vi "Configure Frequency Sweep at Constant Amplitude.vi"(0 "template configuration":refnum<class "SV Signal.lvclass">, 1 "amplitude":dbl=1.0, 5 "frequency range [Hz]":cluster{"start":dbl, "stop":dbl}={"start"=10.0, "stop"=10000.0} {"stop" format="%.2f"; "start" format="%.2f"}, 7 "number of steps":i32=100 min=1, 9 "profile":enum16{"Linear", "Logarithmic"}(ring)=enum."Logarithmic", 11 "error in (no error)":errorcluster) -> (4 "signal configuration":refnum<class "SV Discrete Sweep.lvclass">, 15 "error out":errorcluster)   [LabVIEW 2017, in "SV Discrete Sweep.lvclass"]
doc: "Configures a user-defined test signal. Wire the outputs to SV Signal (waveform) VI to generate the test signal, or wire to SV Signal Property Node to configure additional parameters before wiring to the SV Signal (waveform) VI."
uses:
  <vilib>/addons/_NISVFA/_Generation/Signal Generation/SV Discrete Sweep/SV Discrete Sweep.lvclass
  C:/Program Files (x86)/National Instruments/LabVIEW 2017/vi.lib/addons/_NISVFA/_Generation/Signal Generation/SV Signal/SV Signal.lvclass
  C:/Program Files (x86)/National Instruments/LabVIEW 2017/vi.lib/addons/_NISVFA/_Generation/Signal Generation/SV Function/SV Function.lvclass
  <vilib>/addons/_NISVFA/_Generation/Signal Generation/SV Signal/SV Signal.lvclass
  <vilib>/addons/_NISVFA/_Generation/Signal Generation/SV Signal/sv_System Timing Model.ctl
  <vilib>/addons/_NISVFA/_Generation/Signal Generation/SV Discrete Sweep/SV Discrete Sweep.lvclass/SV Discrete Sweep.ctl
  <vilib>/addons/_NISVFA/_Generation/Signal Generation/SV Signal/Write System Timing Model.vi
  <vilib>/addons/_NISVFA/_Generation/Signal Generation/SV Function/Write Measurement Cycles.vi
  <vilib>/addons/_NISVFA/_Generation/Signal Generation/SV Signal/Write Sample Rate.vi
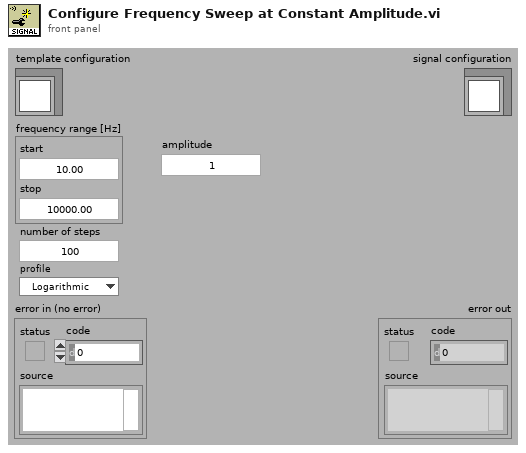
[diagram p1: front panel]
types:
  T1 = cluster{"start frequency":dbl, "stop frequency":dbl, "number of steps":i32}
  T2 = typedef "SV Signal.lvclass/sv_System Timing Model.ctl" = i64
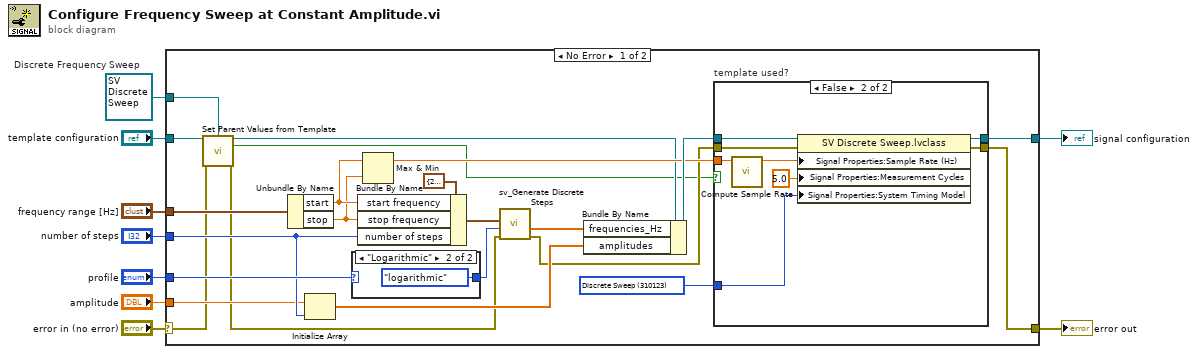
[diagram p0: block diagram]
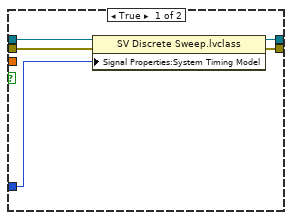
[diagram p2: hidden frame]
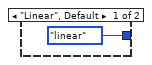
[diagram p3: hidden frame]
diagram:
  w7 = refnum<class "SV Discrete Sweep.lvclass"> refnum  # Discrete Frequency Sweep
  n1 = case shown="No Error" "error in (no error)" {
    selector: "error in (no error)" -> [w12 w48]
    tunnel: [w19 w48] -> w8
    tunnel: [w24 w49] -> w6
    tunnel: w7 -> [w14 w49]
    tunnel: "frequency range [Hz]" -> [w32 _]
    tunnel: "number of steps" -> [w27 _]
    tunnel: "profile" -> [w29 _]
    tunnel: "amplitude" -> [w23 _]
    tunnel: "template configuration" -> [w15 _]
    frame No Error {
      w17 = T2 310123 items=["Finite"=10178, "-"=-1, "Continuous"=10123, "-"=-2, "Settled"=110123, "Averaged"=210123, "Discrete Sweep"=310123, "Continuous Sweep"=410123] ("System Timing Model")
      n2 = call-dynamic "Set Parent Values from Template.vi"("template configuration"=w15, "signal configuration in"=w14, "error in (no error)"=w12) -> ("signal configuration out"=w13:refnum<class "SV Discrete Sweep.lvclass">, "template used?"=w10:bool, "error out"=w11:errorcluster)  [unwired: 10 in]
      n3 = Unbundle By Name(w32) -> ("start"=w22:dbl, "stop"=w21:dbl)
      n4 = Initialize Array(w23, w27) -> (w26:dbl[])
      n5 = case shown="\"Logarithmic\"" w29 {
        tunnel: [enum16{"linear", "logarithmic"}."linear" ("frequency spacing") enum16{"linear", "logarithmic"}."logarithmic" ("frequency spacing")] -> w28
        frame "Linear", Default {
        }
        frame "Logarithmic" {
        }
      }
      n6 = Bundle By Name(cluster=T1 {"start frequency"=20.0, "stop frequency"=20000.0, "number of steps"=100} ("sweep frequencies"), "start frequency"=w22, "stop frequency"=w21, "number of steps"=w27) -> (w30:T1)
      n7 = Max & Min(x=w22, y=w21) -> (max(x,y)=w20:dbl)  [unwired: 1 out]
      n8 = call <vilib>:"sv_Generate Discrete Steps.vi"("error in (no error)"=w11, "spacing"=w28, "steps"=w30) -> ("error out"=w18:errorcluster, "frequency list"=w16:dbl[])  [unwired: 7 in]
      n9 = Bundle By Name(cluster=w13, "frequencies_Hz"=w16, "amplitudes"=w26) -> (w25:refnum<class "SV Discrete Sweep.lvclass">)
      n10 = case "template used?" shown="False" w10 {
        tunnel: w25 -> [w37 w44]
        tunnel: [w36 w43] -> w24
        tunnel: w20 -> [_ w42]
        tunnel: [w35 w41] -> w19
        tunnel: w18 -> [w34 w40]
        tunnel: w17 -> [w33 w39]
        frame True {
          n11 = property class="SV Discrete Sweep.lvclass"(reference=w37, error in=w34, "Signal Properties:System Timing Model"=w33) -> (reference out=w36:refnum<class "SV Discrete Sweep.lvclass">, error out=w35:errorcluster)
        }
        frame False {
          n12 = call <vilib>:"Compute Sample Rate.vi"("maximum frequency [Hz]"=w42) -> ("sample rate [Hz]"=w38:dbl)  [unwired: 10 in]
          n13 = property class="SV Discrete Sweep.lvclass"(reference=w44, error in=w40, "Signal Properties:Sample Rate (Hz)"=w38, "Signal Properties:Measurement Cycles"=5.0 ("Measurement Cycles"), "Signal Properties:System Timing Model"=w39) -> (reference out=w43:refnum<class "SV Discrete Sweep.lvclass">, error out=w41:errorcluster)
        }
      }
    }
    frame Error {
    }
  }
  "error out" <- w8
  "signal configuration" <- w6
